vi "Write Results.vi"(8 "error in (no error)":errorcluster, 10 "Results":refnum<class "Mag Lab Result.lvclass">[](array[class]), 11 "Compound Measurement in":refnum<class "Compound Measurement.lvclass">) -> (0 "error out":errorcluster, 3 "Compound Measurement out":refnum<class "Compound Measurement.lvclass">)   [LabVIEW 2015, in "Compound Measurement.lvclass"]
uses:
  Compound Measurement.lvclass
  Mag Lab Result/Mag Lab Result.lvclass
  Compound Measurement.lvclass/Compound Measurement.ctl
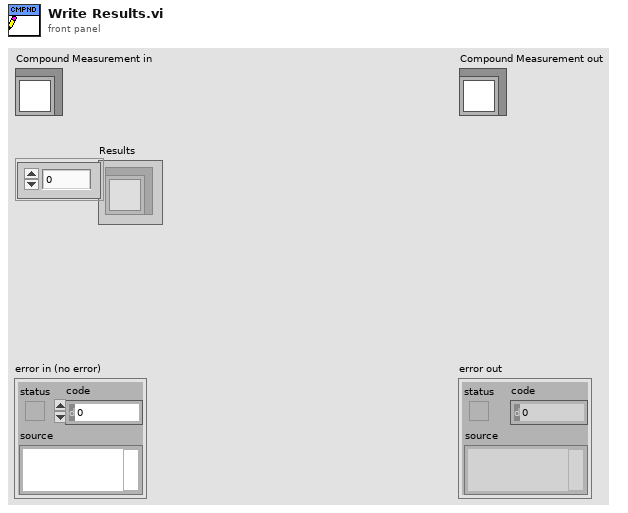
[diagram p1: front panel]
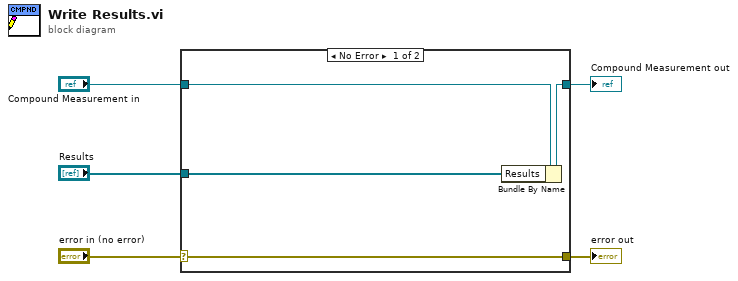
[diagram p0: block diagram]
diagram:
  n1 = case shown="No Error" "error in (no error)" {
    selector: "error in (no error)" -> [w9 w10]
    tunnel: [w9 w10] -> w4
    tunnel: [w7 w11] -> w2
    tunnel: "Compound Measurement in" -> [w8 w11]
    tunnel: "Results" -> [w6 _]
    frame No Error {
      n2 = Bundle By Name(cluster=w8, "Results"=w6) -> (w7:refnum<class "Compound Measurement.lvclass">)
    }
    frame Error {
    }
  }
  "error out" <- w4
  "Compound Measurement out" <- w2
